vi "ActionEngine M1.vi"(5 "ChannelNumber":i32, 7 "Settings":T2={"Step Size (mm)"=10.0, "Initial Position"=0.0, "Move Absolute/Relative Position"=0.0, "Step Delay (ms)"=0, "Velocity (mm/s)"=0.0, "Acceleration (mm/s^2)"=0.0} {"Step Size (mm)" min=0.00046 format="%.8f"}, 8 "SerialNumber":string="26004239", 9 "KCubeStepperControl":refnum<k24>(container), 10 "Action":T3) -> (0 "error out":errorcluster, 2 "Current Position":dbl)   [LabVIEW 2022 SP3]
uses:
  C:/Users/mnopl/OneDrive/Documents/PhiThetaScanning/Thorlabs.MotionControl.Controls.dll
  Thorlabs.MotionControl.Controls.dll
  ActionEngineEnum.ctl
  C:/Users/mnopl/OneDrive/Documents/PhiThetaScanning/Thorlabs.MotionControl.KCube.StepperMotorCLI.dll
  Thorlabs.MotionControl.KCube.StepperMotorCLI.dll
panel:
  out "Settings":T1
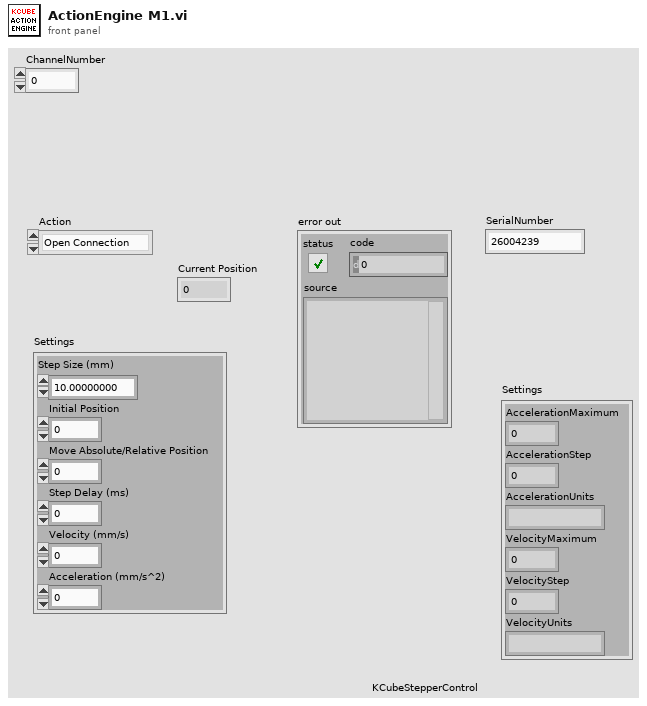
[diagram p1: front panel]
types:
  T1 = cluster{"AccelerationMaximum":dbl, "AccelerationStep":dbl, "AccelerationUnits":string, "VelocityMaximum":dbl, "VelocityStep":dbl, "VelocityUnits":string}
  T2 = cluster{"Step Size (mm)":sgl, "Initial Position":dbl, "Move Absolute/Relative Position":dbl, "Step Delay (ms)":u32, "Velocity (mm/s)":dbl, "Acceleration (mm/s^2)":dbl}
  T3 = typedef "ActionEngineEnum.ctl" = enum16{"Open Connection", "Done", "Get Position", "Settings", "Home", "Move Absolute", "Move Relative", "Step", "Stop Action", "Close Connection"}
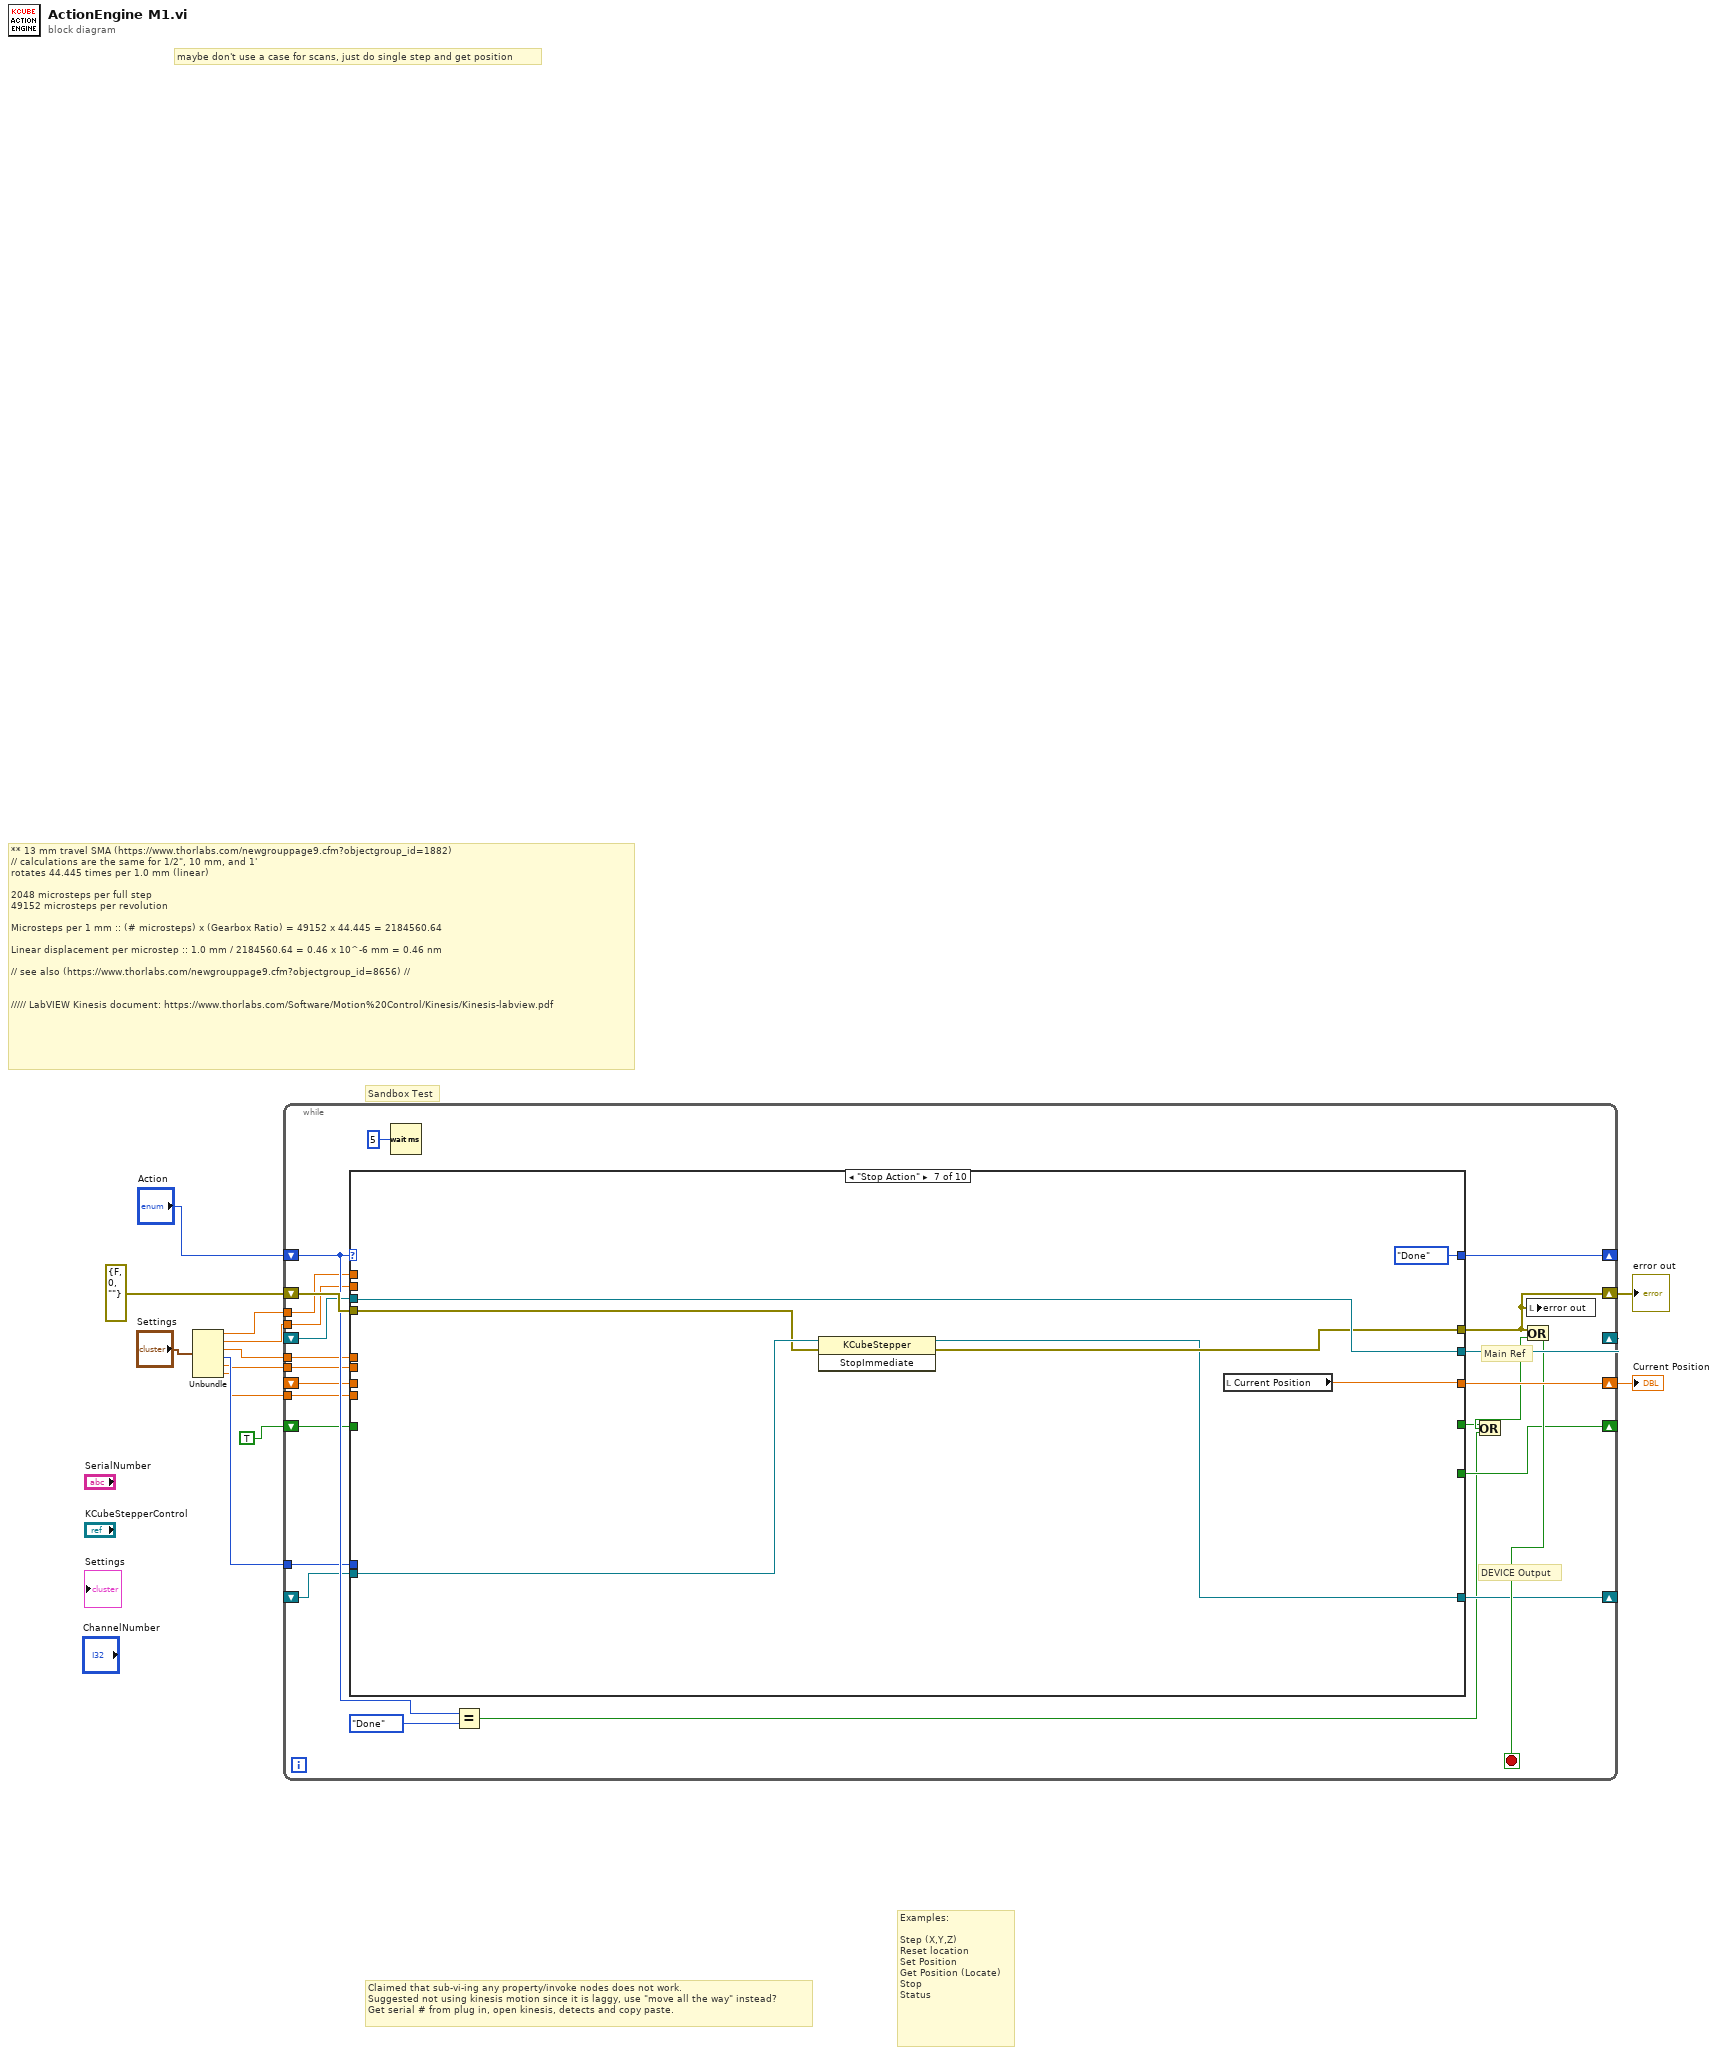
[diagram p0: block diagram]
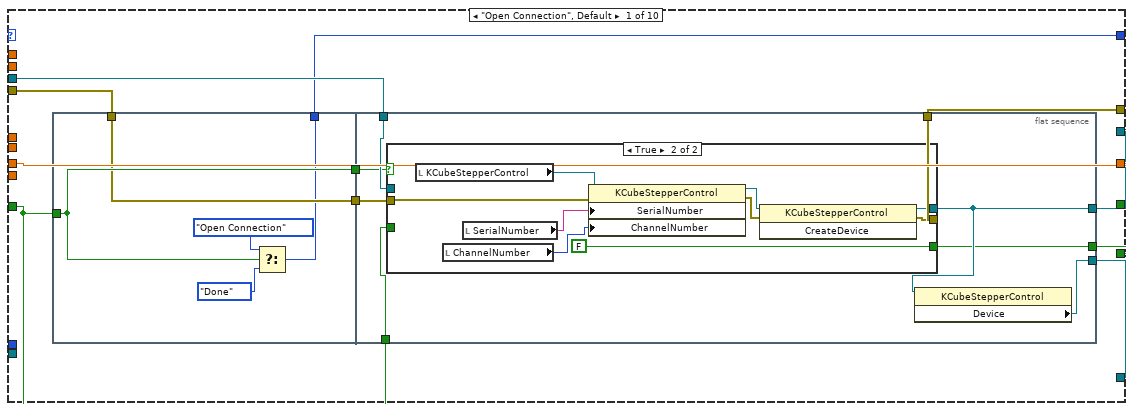
[diagram p2: hidden frame]
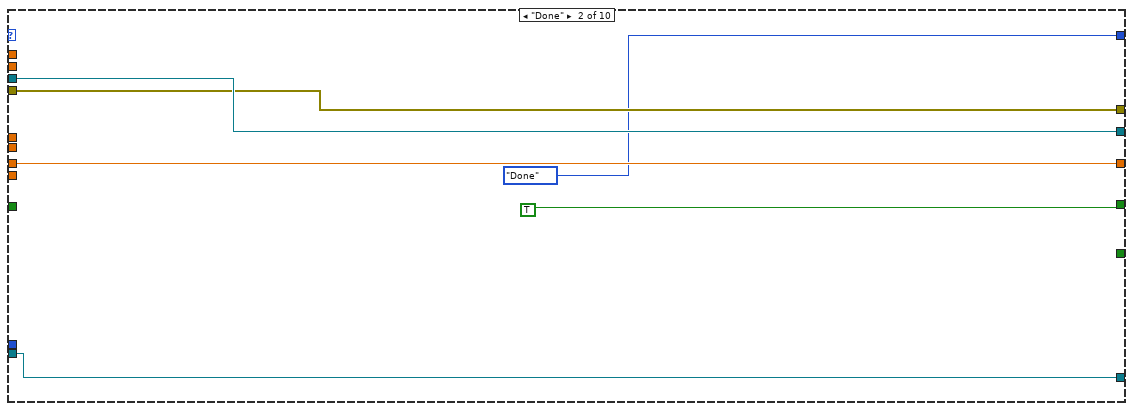
[diagram p4: hidden frame]
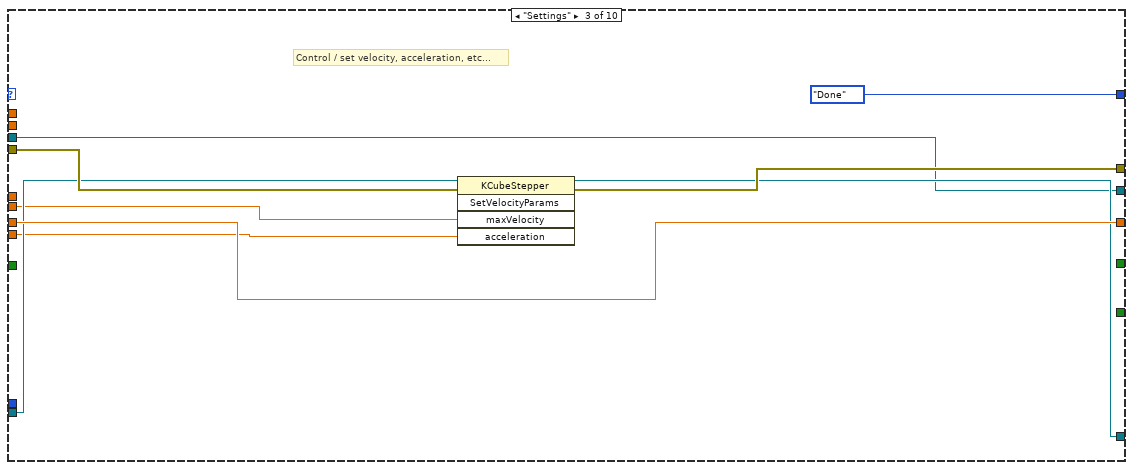
[diagram p5: hidden frame]
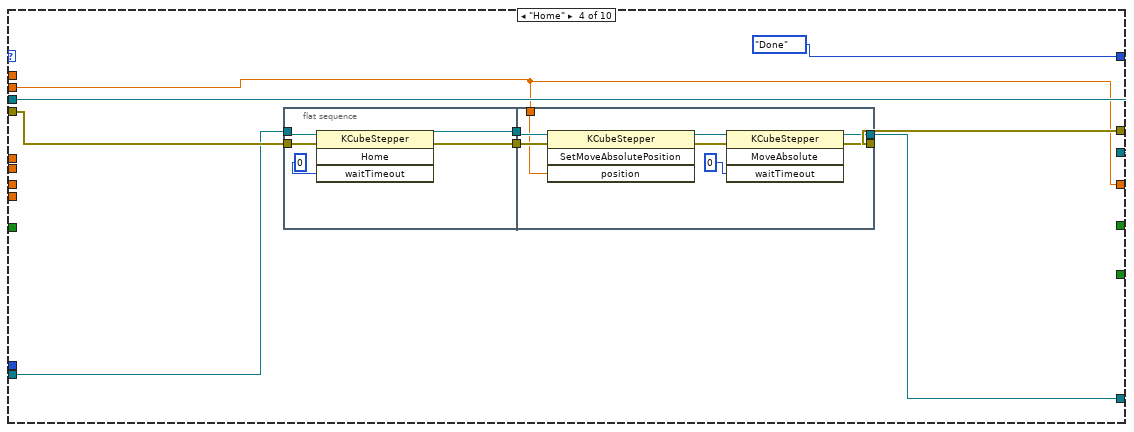
[diagram p6: hidden frame]
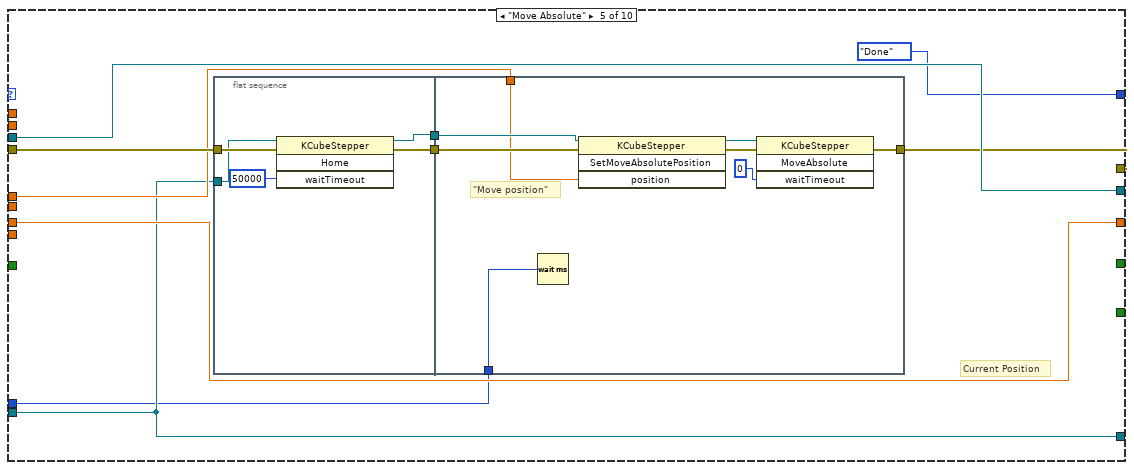
[diagram p7: hidden frame]
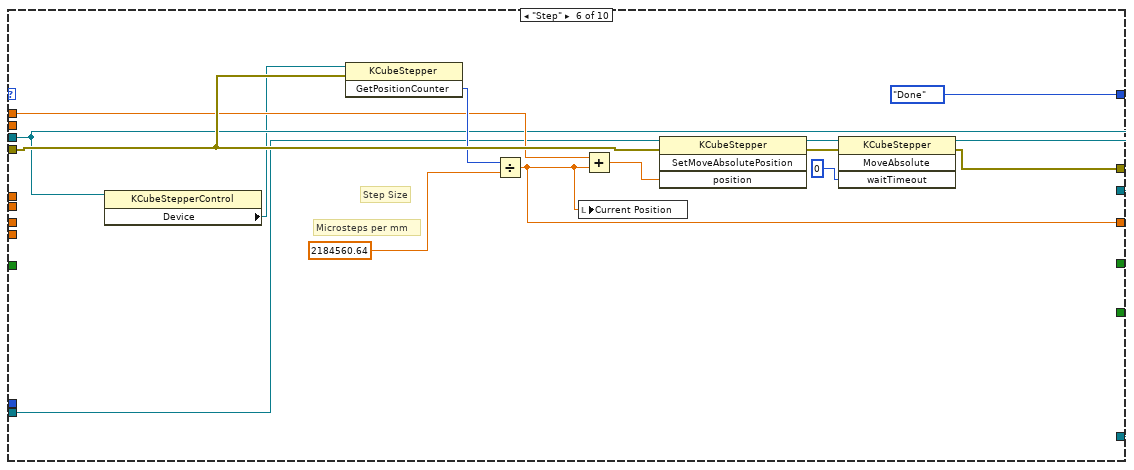
[diagram p8: hidden frame]
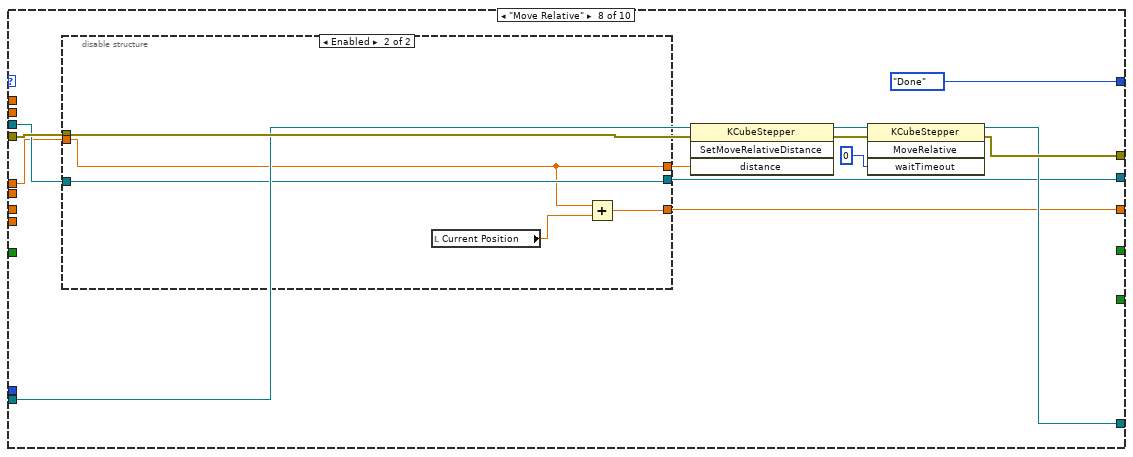
[diagram p9: hidden frame]
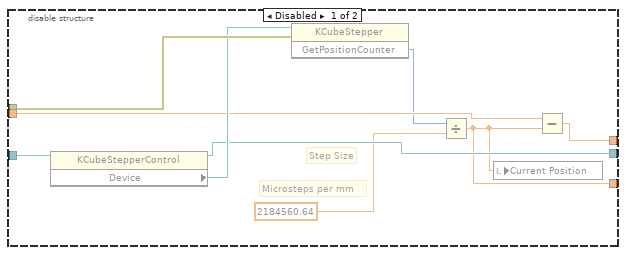
[diagram p10: hidden frame]
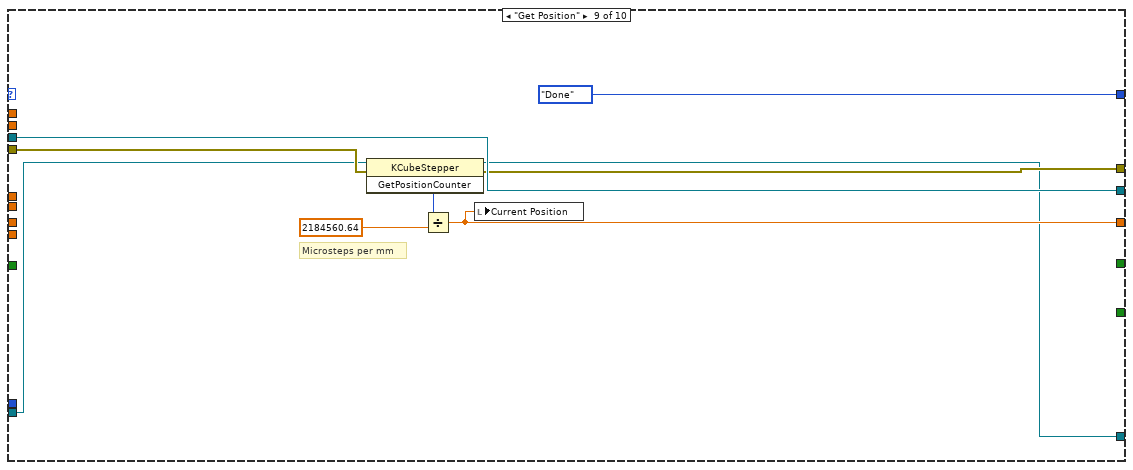
[diagram p11: hidden frame]
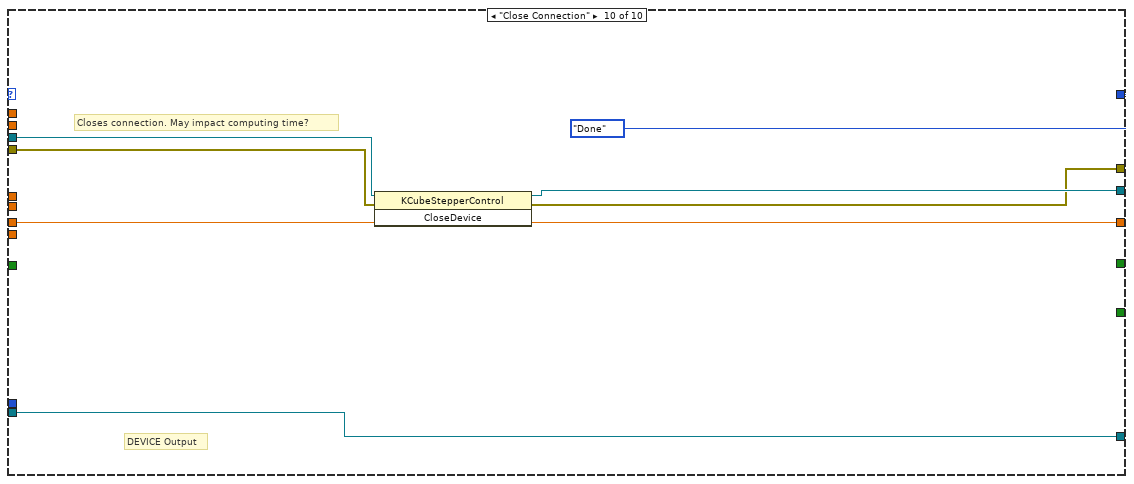
[diagram p12: hidden frame]
diagram:
  # "Claimed that sub-vi-ing any property/invoke nodes does not work.\nSuggested not using kinesis motion since it is laggy, use \"move all the way\" instead?\nGet serial # from plug in, open kinesis, detects and copy paste."
  # "maybe don't use a case for scans, just do single step and get position"
  # "Examples:\n\nStep (X,Y,Z)\nReset location\nSet Position\nGet Position (Locate) \nStop\nStatus"
  # "** 13 mm travel SMA (https://www.thorlabs.com/newgrouppage9.cfm?objectgroup_id=1882)\n// calculations are the same for 1/2\", 10 mm, and 1'\nrotates 44.445 times per 1.0 mm (linear)\n\n2048 microsteps per full step\n49152 microsteps per revolution\n\nMicrosteps per 1 mm :: (# microsteps) x (Gearbox Ratio) = 49152 x 44.445 = 2184560.64\n\nLinear displacement per microstep :: 1.0 mm / 2184560.64 = 0.46 x 10^-6 mm = 0.46 nm\n\n// see also (https://www.thorlabs.com/newgrouppage9.cfm?objectgroup_id=8656) //\n\n\n///// LabVIEW Kinesis document: https://www.thorlabs.com/Software/Motion%20Control/Kinesis/Kinesis-labview.pdf"
  # "Sandbox Test"
  n1 = Unbundle("Settings") -> ("Step Size (mm)"=w9:sgl, "Initial Position"=w10:dbl, "Move Absolute/Relative Position"=w4:dbl, "Step Delay (ms)"=w3:u32, "Velocity (mm/s)"=w2:dbl, "Acceleration (mm/s^2)"=w1:dbl)
  n2 = while {
    shift-right: [w25] -> w12
    shift-left: errorcluster {"status"=FALSE, "code"=0, "source"=""} ("error out") -> [w36]
    shift-right: [w34] -> _
    shift-left: _ -> [w35]
    shift-right: [w32] -> _
    shift-left: "Action" -> [w33]
    tunnel: w10 -> [w30]
    tunnel: w9 -> [w29]
    tunnel: w4 -> [w28]
    shift-right: [w27] -> w8
    shift-left: _ -> [w26]
    shift-right: [w23] -> _
    shift-left: _ -> [w22]
    shift-right: [w20] -> _
    shift-left: TRUE -> [w21]
    tunnel: w3 -> [w16]
    tunnel: w2 -> [w15]
    tunnel: w1 -> [w14]
    stop <- w24 stop-if-true
    # "DEVICE Output"
    # "Main Ref"
    n3 = case shown="\"Stop Action\"" w33 {
      tunnel: w36 -> [w46 w76 w85 w92 w119 w144 w153 w164 w188 w194]
      tunnel: [w43 w76 w84 w93 w112 w143 w151 w163 w185 w190] -> w25
      tunnel: w35 -> [w45 w77 w79 w96 w116 w134 w152 w160 w189 w192]
      tunnel: [w38 w77 w79 w96 w116 w134 w152 w158 w189 w191] -> w34
      tunnel: [w39 ActionEngineEnum."Done" ("Action") ActionEngineEnum."Done" ("Enum") ActionEngineEnum."Done" ("Enum") ActionEngineEnum."Done" ("Enum") ActionEngineEnum."Done" ("Enum") ActionEngineEnum."Done" ("Enum") ActionEngineEnum."Done" ("Enum") ActionEngineEnum."Done" ("Enum") ActionEngineEnum."Done" ("Enum")] -> w32
      tunnel: w30 -> [_ _ _ w88 _ _ _ _ _ _]
      tunnel: w29 -> [_ _ _ _ _ w139 _ _ _ _]
      tunnel: w28 -> [_ _ _ _ w115 _ _ w157 _ _]
      tunnel: [w47 w78 w87 w88 w114 w138 w149 w156 w183 w195] -> w27
      tunnel: w26 -> [w47 w78 w87 _ w114 _ _ _ _ w195]
      tunnel: [w37 w75 w80 w90 w113 w136 w150 w159 w181 w193] -> w23
      tunnel: w22 -> [_ w75 w83 w91 w113 w135 w154 w161 w182 w193]
      tunnel: w21 -> [w44 _ _ _ _ _ _ _ _ _]
      tunnel: [w41 _ _ _ _ _ _ _ _ _] -> w20
      tunnel: [_ TRUE _ _ _ _ _ _ _ _] -> w17
      tunnel: w16 -> [_ _ _ _ w110 _ _ _ _ _]
      tunnel: w15 -> [_ _ w82 _ _ _ _ _ _ _]
      tunnel: w14 -> [_ _ w81 _ _ _ _ _ _ _]
      frame "Open Connection", Default {
        n4 = flat-sequence {
          tunnel: w44 -> [w52]
          tunnel: w46 -> [w49]
          tunnel: [w49] -> w42
          tunnel: [w52] -> w40
          tunnel: [w48] -> w39
          tunnel: w45 -> [w60]
          tunnel: w44 -> [w59]
          tunnel: [w53] -> w37
          tunnel: [w58] -> w43
          tunnel: [w56] -> w38
          tunnel: w42 -> [w57]
          tunnel: [w55] -> w41
          tunnel: w40 -> [w54]
          frame #0 {
            n5 = Select(t=ActionEngineEnum."Open Connection" ("Enum"), s=w52, f=ActionEngineEnum."Done" ("Enum")) -> (s? t:f=w48:T3)
          }
          frame #1 {
            n6 = case shown="True" w54 {
              selector: w54 -> [w61 _]
              tunnel: [w63 w70] -> w58
              tunnel: w57 -> [w63 w72]
              tunnel: [w62 w71] -> w56
              tunnel: w60 -> [w62 _]
              tunnel: w59 -> [_ _]
              tunnel: [w61 FALSE] -> w55
              frame False {
              }
              frame True {
                n7 = local read "KCubeStepperControl"() -> (w67:refnum<k24>)
                n8 = local read "ChannelNumber"() -> (w64:i32)
                n9 = local read "SerialNumber"() -> (w66:string)
                n10 = property class="KCubeStepperControl"(reference=w67, error in=w72, "SerialNumber"=w66, "ChannelNumber"=w64) -> (reference out=w69:refnum<k24>, error out=w68:errorcluster)
                n11 = invoke class="KCubeStepperControl" method="CreateDevice"(reference=w69, error in=w68) -> (reference out=w71:refnum<k24>, error out=w70:errorcluster)  [unwired: 1 in, 1 out]
              }
            }
            n12 = property class="KCubeStepperControl"(reference=w56) -> ("Device"=w53:refnum<k24>)  [unwired: 1 in, 2 out]
          }
        }
      }
      frame "Done" {
      }
      frame "Settings" {
        # "Control / set velocity, acceleration, etc..."
        n13 = invoke class="KCubeStepper" method="SetVelocityParams"(reference=w83, error in=w85, "maxVelocity"=w82, "acceleration"=w81) -> (reference out=w80:refnum<k24>, error out=w84:errorcluster)  [unwired: 1 in, 3 out]
      }
      frame "Home" {
        n14 = flat-sequence {
          tunnel: w91 -> [w101]
          tunnel: w92 -> [w99]
          tunnel: [w98] -> w95
          tunnel: [w97] -> w94
          tunnel: w95 -> [w109]
          tunnel: w94 -> [w108]
          tunnel: [w104] -> w93
          tunnel: w88 -> [w103]
          tunnel: [w102] -> w90
          frame #0 {
            n15 = invoke class="KCubeStepper" method="Home"(reference=w101, error in=w99, "waitTimeout"=0) -> (reference out=w98:refnum<k24>, error out=w97:errorcluster)  [unwired: 1 in, 2 out]
          }
          frame #1 {
            n16 = invoke class="KCubeStepper" method="SetMoveAbsolutePosition"(reference=w109, error in=w108, "position"=w103) -> (reference out=w106:refnum<k24>, error out=w107:errorcluster)  [unwired: 1 in, 2 out]
            n17 = invoke class="KCubeStepper" method="MoveAbsolute"(reference=w106, error in=w107, "waitTimeout"=0) -> (reference out=w102:refnum<k24>, error out=w104:errorcluster)  [unwired: 1 in, 2 out]
          }
        }
      }
      frame "Move Absolute" {
        # "Current Position"
        n18 = flat-sequence {
          tunnel: w113 -> [w120]
          tunnel: w119 -> [w121]
          tunnel: [w123] -> w118
          tunnel: [w122] -> w117
          tunnel: w118 -> [w132]
          tunnel: w117 -> [w131]
          tunnel: [w130] -> w112
          tunnel: w115 -> [w126]
          tunnel: w110 -> [w125]
          frame #0 {
            n19 = invoke class="KCubeStepper" method="Home"(reference=w120, error in=w121, "waitTimeout"=50000) -> (reference out=w123:refnum<k24>, error out=w122:errorcluster)  [unwired: 1 in, 2 out]
          }
          frame #1 {
            # "\"Move position\""
            n20 = Wait (ms)(milliseconds to wait=w125) -> ()  [unwired: 1 out]
            n21 = invoke class="KCubeStepper" method="SetMoveAbsolutePosition"(reference=w132, error in=w131, "position"=w126) -> (reference out=w128:refnum<k24>, error out=w129:errorcluster)  [unwired: 1 in, 2 out]
            n22 = invoke class="KCubeStepper" method="MoveAbsolute"(reference=w128, error in=w129, "waitTimeout"=0) -> (error out=w130:errorcluster)  [unwired: 1 in, 3 out]
          }
        }
      }
      frame "Step" {
        # "Step Size"
        # "Microsteps per mm"
        n23 = property class="KCubeStepperControl"(reference=w134) -> ("Device"=w133:refnum<k24>)  [unwired: 1 in, 2 out]
        n24 = invoke class="KCubeStepper" method="GetPositionCounter"(reference=w133, error in=w144) -> ("GetPositionCounter"=w142:i32)  [unwired: 1 in, 2 out]
        n25 = Divide(x=w142, y=2184560.64) -> (x/y=w138:dbl)
        n26 = local write "Current Position"(w138) -> ()
        n27 = Add(x=w139, y=w138) -> (x+y=w140:dbl)
        n28 = invoke class="KCubeStepper" method="SetMoveAbsolutePosition"(reference=w135, error in=w144, "position"=w140) -> (reference out=w146:refnum<k24>, error out=w147:errorcluster)  [unwired: 1 in, 2 out]
        n29 = invoke class="KCubeStepper" method="MoveAbsolute"(reference=w146, error in=w147, "waitTimeout"=0) -> (reference out=w136:refnum<k24>, error out=w143:errorcluster)  [unwired: 1 in, 2 out]
      }
      frame "Stop Action" {
        n30 = invoke class="KCubeStepper" method="StopImmediate"(reference=w154, error in=w153) -> (reference out=w150:refnum<k24>, error out=w151:errorcluster)  [unwired: 1 in, 1 out]
        n31 = local read "Current Position"() -> (w149:dbl)
      }
      frame "Move Relative" {
        n32 = disable-structure shown="Enabled" {
          disable-tunnel: w164 -> [w176 _]
          disable-tunnel: w160 -> [w175 w180]
          disable-tunnel: [w173 w180] -> w158
          disable-tunnel: w157 -> [w172 w179]
          disable-tunnel: [w171 w177] -> w156
          disable-tunnel: [w170 w179] -> w155
          frame Disabled {
            # "Step Size"
            # "Microsteps per mm"
            n33 = property class="KCubeStepperControl"(reference=w175) -> (reference out=w173:refnum<k24>, "Device"=w174:refnum<k24>)  [unwired: 1 in, 1 out]
            n34 = invoke class="KCubeStepper" method="GetPositionCounter"(reference=w174, error in=w176) -> ("GetPositionCounter"=w169:i32)  [unwired: 1 in, 2 out]
            n35 = Divide(x=w169, y=2184560.64) -> (x/y=w171:dbl)
            n36 = local write "Current Position"(w171) -> ()
            n37 = Subtract(x=w172, y=w171) -> (x-y=w170:dbl)
          }
          frame Enabled {
            n38 = local read "Current Position"() -> (w178:dbl)
            n39 = Add(x=w179, y=w178) -> (x+y=w177:dbl)
          }
        }
        n40 = invoke class="KCubeStepper" method="SetMoveRelativeDistance"(reference=w161, error in=w164, "distance"=w155) -> (reference out=w166:refnum<k24>, error out=w167:errorcluster)  [unwired: 1 in, 2 out]
        n41 = invoke class="KCubeStepper" method="MoveRelative"(reference=w166, error in=w167, "waitTimeout"=0) -> (reference out=w159:refnum<k24>, error out=w163:errorcluster)  [unwired: 1 in, 2 out]
      }
      frame "Get Position" {
        # "Microsteps per mm"
        n42 = invoke class="KCubeStepper" method="GetPositionCounter"(reference=w182, error in=w188) -> (reference out=w181:refnum<k24>, error out=w185:errorcluster, "GetPositionCounter"=w187:i32)  [unwired: 1 in]
        n43 = Divide(x=w187, y=2184560.64) -> (x/y=w183:dbl)
        n44 = local write "Current Position"(w183) -> ()
      }
      frame "Close Connection" {
        # "DEVICE Output"
        # "Closes connection. May impact computing time?"
        n45 = invoke class="KCubeStepperControl" method="CloseDevice"(reference=w192, error in=w194) -> (reference out=w191:refnum<k24>, error out=w190:errorcluster)  [unwired: 1 in, 1 out]
      }
    }
    n46 = Wait (ms)(milliseconds to wait=u32 5) -> ()  [unwired: 1 out]
    n47 = Equal?(x=w33, y=ActionEngineEnum."Done" ("Enum")) -> (x = y?=w18:bool)
    n48 = Or(x=w17, y=w18) -> (x .or. y?=w19:bool)
    n49 = Or(x=w25, y=w19) -> (x .or. y?=w24:bool)
    n50 = local write "error out"(w25) -> ()
  }
  "error out" <- w12
  "Current Position" <- w8
